vi "WriteImageFileTIFF.vi"(7 "Color Palette":T2[](array[typedef]), 8 "error in":errorcluster, 9 "TIFF Options":T1={"Rows Per Strip"=0.0, "Photometric"=1, "Compression Type"=0} {"Compression Type" items=["None", "JPEG", "Run Length Encoded", "Zip"]; "Photometric" items=["WhiteIsZero", "BlackIsZero"]}, 10 "File Path":path, 11 "Image Reference In":T3) -> (0 "error out":errorcluster, 3 "Image Reference Out":T3)   [LabVIEW 2024, in "OpenLvVision_Image.lvlib" / "File.lvlib"]
doc: "Saves the image to a file in the chosen format."
uses:
  File.lvlib
  Management/TypeDef/Image.ctl
  TypeDef/ColorPaletteValue.ctl
  TypeDef/TiffOptions.ctl
  Management/Management.lvlib
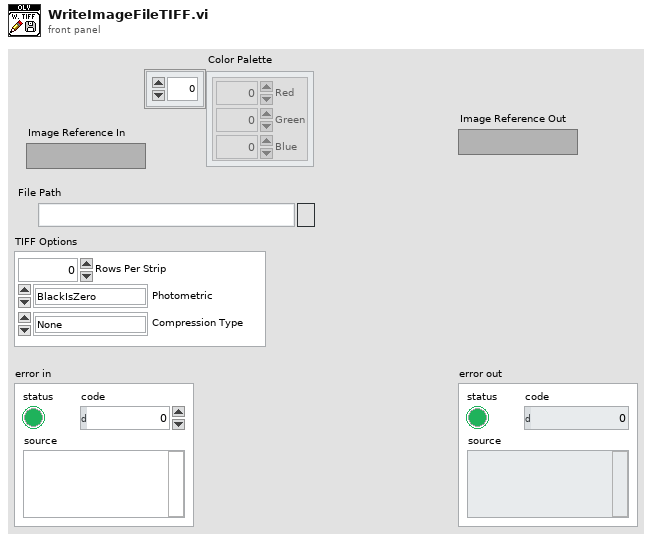
[diagram p1: front panel]
types:
  T1 = typedef "OpenLvVision_Image.lvlib/File.lvlib/TiffOptions.ctl" = cluster{"Rows Per Strip":dbl, "Photometric":i32, "Compression Type":i32}
  T2 = typedef "OpenLvVision_Image.lvlib/File.lvlib/ColorPaletteValue.ctl" = cluster{"Red":u8, "Green":u8, "Blue":u8}
  T3 = typedef "OpenLvVision_Image.lvlib/Management.lvlib/Image.ctl" = refnum<image>
  T4 = typedef "IMAQ Image.ctl" = refnum<image>
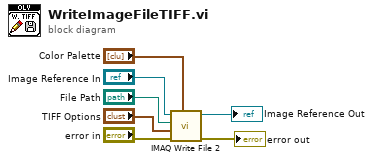
[diagram p0: block diagram]
diagram:
  n1 = call-poly "IMAQ Write File 2"("Color Palette"="Color Palette", "error in (no error)"="error in", "TIFF Options"="TIFF Options", "File Path"="File Path", "Image"="Image Reference In") -> ("error out"=→"error out":errorcluster, "Image Out (duplicate)"=→"Image Reference Out":T4)  [unwired: 5 in]
